vi "main_copy.vi"() -> ()   [LabVIEW 2017]
uses:
  <vilib>/DAQmx/write.llb/DAQmx Write (Digital Bool 1Line 1Point).vi
  <vilib>/DAQmx/read.llb/DAQmx Read (Counter U32 1Chan 1Samp).vi
  <vilib>/DAQmx/write.llb/DAQmx Write (Digital 1D Bool 1Chan 1Samp).vi
  <vilib>/DAQmx/create/channels.llb/DAQmx Create Channel (CI-Count Edges).vi
  <vilib>/DAQmx/miscellaneous.llb/DAQmx Fill In Error Info.vi
  <vilib>/DAQmx/create/channels.llb/DAQmx Create Channel (DO-Digital Output).vi
  <resource>/objmgr/daqmx.rc
panel:
  in  "Digital real/sham stim channels":tag="PCI-DAQ/port0/line3, PCI-DAQ/port0/line7"
  in  "Analog pulse channel":tag="PCI-DAQ/ao0"
  in  "OEP sample clock in":tag="/PCI-DAQ/PFI0"
  in  "Onboard counter":tag="PCI-DAQ/ctr1"
  in  "DAQ probe channel":tag="PCI-DAQ/port0/line5"
  out "Learning rate (for adaptive threshold)":dbl(graph)=0.005000000792214087
  out "Phase threshold":sgl(graph)=145.96965
  in  "Stim even when\ntarget exceeded":bool=TRUE
  in  "Sham stimulations:":i32=1 min=0
  in  "Real stimulations:":i32=1 min=1
  out "Stim time":i64
  out "Crossing time":i64
  out "Crossing level":sgl
  out "Time on (samp.)":i64
  out "Clock offset":i64
  in  "probe channel":u16=8 min=1 max=8
  in  "event channel":u16=5 min=1 max=8
  in  "event port":u16=5558
  out "New event":bool
  in  "Max target":i64 min=0
  in  "Limit target":bool
  in  "Target delay":i64
  in  "Adapt target":bool
  out "Phase offset (deg.)":dbl
  in  "Avg signal freq (Hz)":dbl=6.0
  in  "Sample rate":dbl=30000.0
  in  "Stim enabled":bool
  out "OEP to LV delay":i64(graph)=235
  in  "Stop":bool
  # "FOR USE WHEN DOING 2 (OR...MORE?) CL TESTS SIMULTANEOUSLY.\nIf there are any major changes to main.vi, make sure to update this copy as well.\nYou can either use this along with main.vi, or make another copy of this with another name, but if you use main.vi, make sure to\ndisable all the analog out stuff as it is in here. Either way you also have to disable the analog out channel creation in PrepareChannels_v2.vi.\nOutputting on 2 analog channels at once with separate sample clocks isn't possible (with our DAQ).\nMake sure other channels also don't conflict between the two instances, except the sample clock in can be the same."
  # "*** Start OpenEphys acquisition before the VI. ***"
  # "*** In the audio settings in the OpenEphys GUI, reduce the buffer size to get a 10 ms buffer period.  If ASIO is installed and enabled in\nthe Open Ephys build, use ASIO with sample rate (in audio settings) = 192,000 Hz and buffer size = 192 (1 ms buffer period). ***"
  # "Inputs"
  # "Delay control"
  # "Stim pattern if enabled"
  # "Event info"
  # "Threshold estimation"
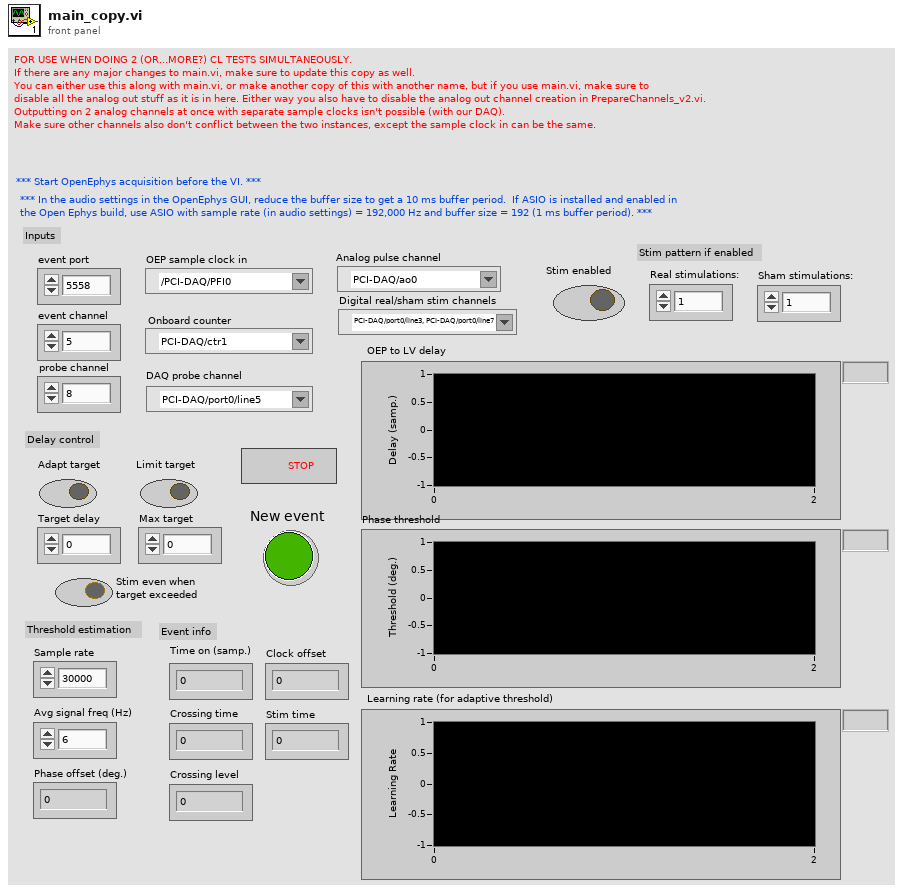
[diagram p1: front panel]
types:
  T1 = typedef "Rendezvous RefNum" = refnum<k1>
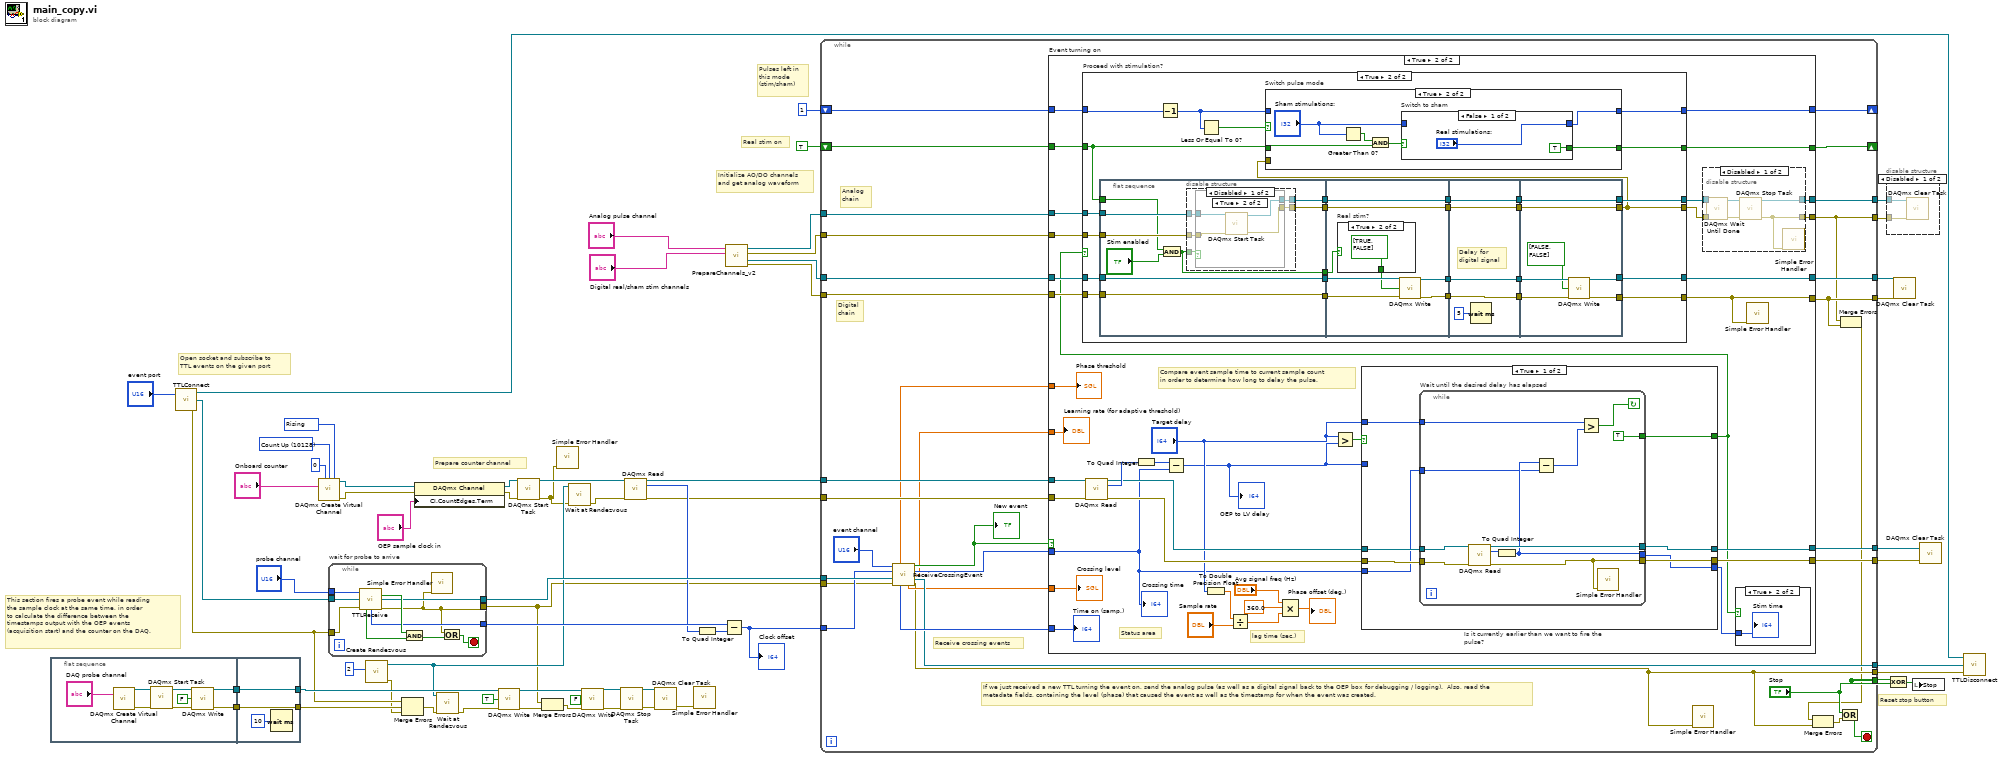
[diagram p0: block diagram]
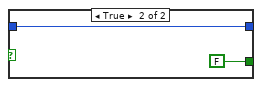
[diagram p8: hidden frame]
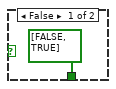
[diagram p11: hidden frame]
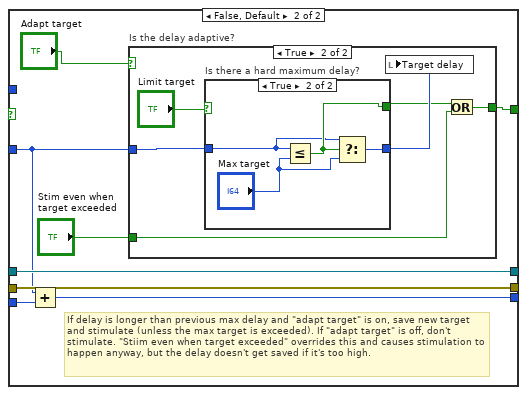
[diagram p12: hidden frame]
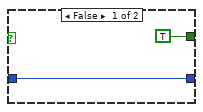
[diagram p14: hidden frame]
diagram:
  w48 = 10280 items=["Rising"=10280, "Falling"=10171] ("edge")
  w49 = 10128 items=["Count Up"=10128, "Count Down"=10124, "Externally Controlled"=10326] ("count direction")
  # "Pulses left in \nthis mode\n(stim/sham)"
  # "Real stim on"
  # "Reset stop button"
  # "This section fires a probe event while reading\nthe sample clock at the same time, in order\nto calculate the difference between the \ntimestamps output with the OEP events\n(acquisition start) and the counter on the DAQ."
  # "Prepare counter channel"
  # "Initialize AO/DO channels\nand get analog waveform"
  # "Open socket and subscribe to\nTTL events on the given port"
  n1 = flat-sequence {
    tunnel: [w66] -> w31
    tunnel: [w64] -> w30
    tunnel: [w72] -> w21
    tunnel: [w73] -> w28
    tunnel: w31 -> [w73]
    tunnel: w30 -> [w72]
    frame #0 {
      n2 = call-poly <vilib>:"DAQmx Create Virtual Channel.vi"("lines"="DAQ probe channel") -> ("task out"=w69:refnum<k21>, "error out"=w70:errorcluster)  [unwired: 13 in]
      n3 = call <vilib>:"DAQmx Start Task.vi"("task/channels in"=w69, "error in"=w70) -> ("task out"=w67:refnum<k21>, "error out"=w65:errorcluster)  [unwired: 12 in]
      n4 = call-poly <vilib>:"DAQmx Write.vi"("task/channels in"=w67, "data"=FALSE, "error in"=w65) -> ("task out"=w66:refnum<k21>, "error out"=w64:errorcluster)  [unwired: 10 in, 1 out]
    }
    frame #1 {
      n5 = Wait (ms)(milliseconds to wait=u32 10) -> ()  [unwired: 1 out]
    }
  }
  n6 = call "TTLConnect.vi"("port"="event port") -> ("context out"=w61:refnum<class "zmq_context.lvclass">, "socket out"=w43:refnum<class "zmq_socket.lvclass">, "error out"=w22:errorcluster)  [unwired: 1 in]
  n7 = call-poly <vilib>:"DAQmx Create Virtual Channel.vi"("initial count"=u32 0, "count direction"=w49, "edge"=w48, "counter"="Onboard counter") -> ("task out"=w51:refnum<k21>, "error out"=w50:errorcluster)  [unwired: 10 in]
  n8 = while "wait for probe to arrive" {
    tunnel: w43 -> [w83]
    tunnel: "probe channel" -> [w82]
    tunnel: [w79] -> w41
    tunnel: [w74] -> w11
    tunnel: [w78] -> w32
    tunnel: w22 -> [w77]
    stop <- w76 stop-if-true
    n9 = call "TTLReceive.vi"("channel"=w82, "socket in"=w83, "error in"=w77) -> ("new TTL"=w81:bool, "socket out"=w78:refnum<class "zmq_socket.lvclass">, "event on"=w80:bool, "timestamp"=w79:i64, "error out"=w74:errorcluster)  [unwired: 6 in, 2 out]
    n10 = And(x=w81, y=w80) -> (x .and. y?=w75:bool)
    n11 = call <vilib>:"Simple Error Handler.vi"("error in (no error)"=w74) -> ()  [unwired: 4 in, 5 out]
    n12 = Or(x=w74, y=w75) -> (x .or. y?=w76:bool)
  }
  n13 = call <vilib>:"Create Rendezvous.vi"("size (2)"=2) -> ("error out"=w14:errorcluster, "rendezvous"=w20:T1)  [unwired: 4 in, 1 out]
  n14 = Merge Errors(w22, w21, w14) -> (w19:errorcluster)
  n15 = property class="DAQmx Channel"(reference=w51, error in=w50, "CI.CountEdges.Term"="OEP sample clock in") -> (reference out=w47:refnum<k21>, error out=w46:errorcluster)
  n16 = call <vilib>:"Wait at Rendezvous.vi"("error in (no error)"=w19, "rendezvous"=w20) -> ("error out"=w18:errorcluster)  [unwired: 3 in, 2 out]
  n17 = call-poly <vilib>:"DAQmx Write.vi"("task/channels in"=w28, "data"=TRUE, "error in"=w18) -> ("task out"=w27:refnum<k21>, "error out"=w17:errorcluster)  [unwired: 10 in, 1 out]
  n18 = call <vilib>:"DAQmx Start Task.vi"("task/channels in"=w47, "error in"=w46) -> ("task out"=w39:refnum<k21>, "error out"=w2:errorcluster)  [unwired: 12 in]
  n19 = Merge Errors(w11, w17) -> (w16:errorcluster)
  n20 = call <vilib>:"Simple Error Handler.vi"("error in (no error)"=w2) -> ()  [unwired: 4 in, 5 out]
  n21 = call <vilib>:"Wait at Rendezvous.vi"("error in (no error)"=w2, "rendezvous"=w20) -> ("error out"=w23:errorcluster)  [unwired: 3 in, 2 out]
  n22 = call-poly <vilib>:"DAQmx Write.vi"("task/channels in"=w27, "data"=FALSE, "error in"=w16) -> ("task out"=w35:refnum<k21>, "error out"=w34:errorcluster)  [unwired: 10 in, 1 out]
  n23 = call <vilib>:"DAQmx Stop Task.vi"("task/channels in"=w35, "error in"=w34) -> ("task out"=w38:refnum<k21>, "error out"=w37:errorcluster)  [unwired: 12 in]
  n24 = call-poly <vilib>:"DAQmx Read.vi"("task/channels in"=w39, "error in"=w23) -> ("task out"=w12:refnum<k21>, "data"=w26:u32, "error out"=w24:errorcluster)  [unwired: 11 in]
  n25 = call <vilib>:"DAQmx Clear Task.vi"("task in"=w38, "error in"=w37) -> ("error out"=w1:errorcluster)  [unwired: 13 in]
  n26 = call <vilib>:"Simple Error Handler.vi"("error in (no error)"=w1) -> ()  [unwired: 4 in, 5 out]
  n27 = To Quad Integer(1:w26) -> (0:w29:i64)
  n28 = Subtract(x=w41, y=w29) -> (x-y=w40:i64)
  "Clock offset" <- w40
  n29 = call "PrepareChannels_v2.vi"("AO Physical channels"="Analog pulse channel", "DO Physical channels"="Digital real/sham stim channels") -> ("AO task out"=w60:refnum<k21>, "AO error out"=w57:errorcluster, "DO task out"=w59:refnum<k21>, "DO error out"=w58:errorcluster)  [unwired: 4 in, 1 out]
  n30 = while {
    tunnel: w11 -> [w103]
    tunnel: [w86] -> w52
    tunnel: w32 -> [w105]
    tunnel: w60 -> [w115]
    tunnel: w59 -> [w114]
    tunnel: w58 -> [w113]
    tunnel: w57 -> [w108]
    tunnel: [w106] -> w4
    tunnel: [w85] -> w3
    tunnel: [w112] -> w56
    tunnel: [w87] -> w55
    tunnel: ["Stop"] -> w54
    tunnel: w12 -> [w111]
    tunnel: [w110] -> w45
    tunnel: [w109] -> w44
    tunnel: w40 -> [w104]
    tunnel: w24 -> [w107]
    tunnel: [w99] -> w13
    shift-right: [w93] -> _
    shift-left: TRUE -> [w95]
    shift-right: [w94] -> _
    shift-left: 1 -> [w96]
    stop <- w90 stop-if-true
    # "Analog \nchain"
    # "Digital\nchain"
    # "If we just received a new TTL turning the event on, send the analog pulse (as well as a digital signal back to the OEP box for debugging / logging).  Also, read the metadata fields, containing the level (phase) that caused the event as well as the timestamp for when the event was created."
    # "Receive crossing events"
    n31 = call "ReceiveCrossingEvent.vi"("channel"="event channel", "clock offset"=w104, "socket in"=w105, "error in"=w103) -> ("threshold"=w92:sgl, "new crossing"=w102:bool, "crossing time"=w101:i64, "learning rate"=w91:dbl, "socket out"=w99:refnum<class "zmq_socket.lvclass">, "event time"=w100:i64, "crossing level"=w98:sgl, "error out"=w86:errorcluster)  [unwired: 3 in, 1 out]
    "New event" <- w102
    n32 = case "Event turning on" shown="True" w102 {
      tunnel: w115 -> [w123 w157]
      tunnel: w108 -> [w122 w156]
      tunnel: [w123 w148] -> w106
      tunnel: [w122 w125] -> w85
      tunnel: w114 -> [w121 w160]
      tunnel: w113 -> [w120 w158]
      tunnel: [w121 w161] -> w112
      tunnel: [w120 w124] -> w87
      tunnel: w101 -> [_ w143]
      tunnel: w111 -> [w119 w155]
      tunnel: w107 -> [w118 w152]
      tunnel: [w119 w150] -> w110
      tunnel: [w118 w149] -> w109
      tunnel: w100 -> [_ w144]
      tunnel: w98 -> [_ w138]
      tunnel: w96 -> [w117 w131]
      tunnel: w95 -> [w116 w130]
      tunnel: [w117 w129] -> w94
      tunnel: [w116 w128] -> w93
      tunnel: w92 -> [_ w127]
      tunnel: w91 -> [_ w126]
      frame False {
      }
      frame True {
        # "Status area"
        # "lag time (sec.)"
        # "Compare event sample time to current sample count\nin order to determine how long to delay the pulse."
        n33 = call-poly <vilib>:"DAQmx Read.vi"("task/channels in"=w155, "error in"=w152) -> ("task out"=w151:refnum<k21>, "data"=w154:u32, "error out"=w153:errorcluster)  [unwired: 11 in]
        n34 = To Quad Integer(1:w154) -> (0:w134:i64)
        n35 = Subtract(x=w134, y=w143) -> (x-y=w145:i64)
        "OEP to LV delay" <- w145
        n36 = To Double Precision Float(number="Target delay") -> (double precision float=w142:dbl)
        n37 = Divide(x=w142, y="Sample rate") -> (x/y=w141:dbl)
        n38 = Compound Arithmetic op=MULTIPLY("Avg signal freq (Hz)", 360.0 ("y"), w141) -> (→"Phase offset (deg.)":dbl)
        n39 = Greater?(x="Target delay", y=w145) -> (0:w159:bool)
        n40 = case "Is it currently earlier than we want to fire the pulse?" shown="True" w159 {
          tunnel: w145 -> [_ w281]
          tunnel: "Target delay" -> [w261 _]
          tunnel: w153 -> [w266 w286]
          tunnel: [w265 w286] -> w149
          tunnel: w143 -> [w260 w284]
          tunnel: w151 -> [w267 w285]
          tunnel: [w264 w285] -> w150
          tunnel: [w263 w280] -> w133
          tunnel: [w262 w283] -> w132
          frame True {
            n41 = while "Wait until the desired delay has elapsed" {
              tunnel: w267 -> [w277]
              tunnel: w266 -> [w278]
              tunnel: [w268] -> w265
              tunnel: [w276] -> w264
              tunnel: [TRUE] -> w263
              tunnel: [w271] -> w262
              tunnel: w261 -> [w272]
              tunnel: w260 -> [w270]
              stop <- w274 continue-if-true
              n42 = call-poly <vilib>:"DAQmx Read.vi"("task/channels in"=w277, "error in"=w278) -> ("task out"=w276:refnum<k21>, "data"=w273:u32, "error out"=w268:errorcluster)  [unwired: 11 in]
              n43 = To Quad Integer(1:w273) -> (0:w271:i64)
              n44 = Subtract(x=w271, y=w270) -> (x-y=w269:i64)
              n45 = Greater?(x=w272, y=w269) -> (0:w274:bool)
              n46 = call <vilib>:"Simple Error Handler.vi"("error in (no error)"=w268) -> ()  [unwired: 4 in, 5 out]
            }
          }
          frame False, Default {
            # "If delay is longer than previous max delay and \"adapt target\" is on, save new target and stimulate (unless the max target is exceeded). If \"adapt target\" is off, don't stimulate. \"Stiim even when target exceeded\" overrides this and causes stimulation to happen anyway, but the delay doesn't get saved if it's too high."
            n47 = Add(x=w281, y=w284) -> (x+y=w283:i64)
            n48 = case "Is the delay adaptive?" shown="True" "Adapt target" {
              tunnel: w281 -> [_ w292]
              tunnel: [w287 w290] -> w280
              tunnel: "Stim even when\ntarget exceeded" -> [w287 w288]
              frame False {
              }
              frame True {
                n49 = case "Is there a hard maximum delay?" shown="True" "Limit target" {
                  tunnel: [w295 w299] -> w291
                  tunnel: w292 -> [w295 w297]
                  tunnel: [TRUE w298] -> w289
                  frame False {
                  }
                  frame True {
                    n50 = Less Or Equal?(x=w297, y="Max target") -> (x <= y?=w298:bool)
                    n51 = Select(t=w297, s=w298, f="Max target") -> (s? t:f=w299:i64)
                  }
                }
                n52 = local write "Target delay"(w291) -> ()
                n53 = Or(x=w289, y=w288) -> (x .or. y?=w290:bool)
              }
            }
          }
        }
        n54 = case "Proceed with stimulation?" shown="True" w133 {
          tunnel: [w174 w191] -> w161
          tunnel: w160 -> [w174 w190]
          tunnel: w158 -> [w173 w189]
          tunnel: w157 -> [w176 w188]
          tunnel: w156 -> [w175 w187]
          tunnel: [w173 w186] -> w124
          tunnel: [w175 w183] -> w135
          tunnel: [w176 w185] -> w147
          tunnel: w131 -> [w172 w182]
          tunnel: w130 -> [w171 w179]
          tunnel: [w172 w178] -> w129
          tunnel: [w171 w177] -> w128
          frame False {
          }
          frame True {
            n55 = flat-sequence {
              tunnel: [w224] -> w203
              tunnel: [w221] -> w202
              tunnel: [w220] -> w201
              tunnel: w189 -> [w220]
              tunnel: w190 -> [w221]
              tunnel: w187 -> [w223]
              tunnel: w188 -> [w222]
              tunnel: [w219] -> w200
              tunnel: w179 -> [w217]
              tunnel: [w216] -> w184
              tunnel: [w243] -> w199
              tunnel: [w241] -> w198
              tunnel: w203 -> [w245]
              tunnel: [w245] -> w197
              tunnel: w202 -> [w244]
              tunnel: w201 -> [w242]
              tunnel: w200 -> [w240]
              tunnel: [w240] -> w196
              tunnel: w184 -> [w239]
              tunnel: [w252] -> w195
              tunnel: w199 -> [w252]
              tunnel: [w251] -> w194
              tunnel: w198 -> [w251]
              tunnel: w197 -> [w249]
              tunnel: [w249] -> w193
              tunnel: w196 -> [w248]
              tunnel: [w248] -> w192
              tunnel: [w258] -> w191
              tunnel: w195 -> [w259]
              tunnel: w194 -> [w257]
              tunnel: [w256] -> w186
              tunnel: w193 -> [w255]
              tunnel: [w255] -> w185
              tunnel: [w254] -> w183
              tunnel: w192 -> [w254]
              frame #0 {
                n56 = And(x=w217, y="Stim enabled") -> (x .and. y?=w216:bool)
                n57 = disable-structure shown="Disabled" {
                  disable-tunnel: [w229 w237] -> w224
                  disable-tunnel: w223 -> [w228 w236]
                  disable-tunnel: w222 -> [w227 w237]
                  disable-tunnel: [w226 w236] -> w219
                  disable-tunnel: w216 -> [w225 _]
                  frame Disabled {
                    n58 = case shown="True" w225 {
                      tunnel: [w231 w235] -> w229
                      tunnel: w228 -> [w230 w234]
                      tunnel: w227 -> [w231 w233]
                      tunnel: [w230 w232] -> w226
                      frame False {
                      }
                      frame True {
                        n59 = call <vilib>:"DAQmx Start Task.vi"("task/channels in"=w233, "error in"=w234) -> ("task out"=w235:refnum<k21>, "error out"=w232:errorcluster)  [unwired: 12 in]
                      }
                    }
                  }
                  frame Enabled {
                  }
                }
              }
              frame #1 {
                n60 = case "Real stim?" shown="True" w239 {
                  tunnel: [bool[] [FALSE, TRUE] ("data") bool[] [TRUE, FALSE] ("data")] -> w238
                  frame False {
                  }
                  frame True {
                  }
                }
                n61 = call-poly <vilib>:"DAQmx Write.vi"("task/channels in"=w244, "data"=w238, "error in"=w242) -> ("task out"=w243:refnum<k21>, "error out"=w241:errorcluster)  [unwired: 10 in, 1 out]
              }
              frame #2 {
                # "Delay for \ndigital signal"
                n62 = Wait (ms)(milliseconds to wait=u32 5) -> ()  [unwired: 1 out]
              }
              frame #3 {
                n63 = call-poly <vilib>:"DAQmx Write.vi"("task/channels in"=w259, "data"=bool[] [FALSE, FALSE], "error in"=w257) -> ("task out"=w258:refnum<k21>, "error out"=w256:errorcluster)  [unwired: 10 in, 1 out]
              }
            }
            n64 = Decrement(x=w182) -> (x-1=w180:i32)
            n65 = Less Or Equal To 0?(x=w180) -> (x <= 0?=w181:bool)
            n66 = case "Switch pulse mode" shown="True" w181 {
              tunnel: w183 -> [_ _]
              tunnel: w180 -> [w205 _]
              tunnel: w179 -> [w204 w210]
              tunnel: [w205 w207] -> w178
              tunnel: [w204 w206] -> w177
              frame False {
              }
              frame True {
                n67 = Greater Than 0?(x="Sham stimulations:") -> (x > 0?=w211:bool)
                n68 = And(x=w211, y=w210) -> (x .and. y?=w209:bool)
                n69 = case "Switch to sham" shown="False" w209 {
                  tunnel: "Sham stimulations:" -> [_ w215]
                  tunnel: ["Real stimulations:" w215] -> w207
                  tunnel: [TRUE FALSE] -> w206
                  frame False {
                  }
                  frame True {
                  }
                }
              }
            }
          }
        }
        n70 = disable-structure shown="Disabled" {
          disable-tunnel: [w165 w169] -> w148
          disable-tunnel: w147 -> [w164 w169]
          disable-tunnel: w135 -> [w163 w168]
          disable-tunnel: [w162 w168] -> w125
          frame Disabled {
            n71 = call <vilib>:"DAQmx Wait Until Done.vi"("task/channels in"=w164, "error in"=w163) -> ("task out"=w166:refnum<k21>, "error out"=w167:errorcluster)  [unwired: 12 in]
            n72 = call <vilib>:"DAQmx Stop Task.vi"("task/channels in"=w166, "error in"=w167) -> ("task out"=w165:refnum<k21>, "error out"=w162:errorcluster)  [unwired: 12 in]
            n73 = call <vilib>:"Simple Error Handler.vi"("error in (no error)"=w162) -> ()  [unwired: 4 in, 5 out]
          }
          frame Enabled {
          }
        }
        n74 = case shown="True" w133 {
          tunnel: w132 -> [_ w170]
          frame False {
          }
          frame True {
            "Stim time" <- w170
          }
        }
        n75 = call <vilib>:"Simple Error Handler.vi"("error in (no error)"=w124) -> ()  [unwired: 4 in, 5 out]
        "Time on (samp.)" <- w144
        "Crossing time" <- w143
        "Crossing level" <- w138
        "Phase threshold" <- w127
        "Learning rate (for adaptive threshold)" <- w126
      }
    }
    n76 = call <vilib>:"Simple Error Handler.vi"("error in (no error)"=w86) -> ()  [unwired: 4 in, 5 out]
    n77 = Merge Errors(w85, w87) -> (w84:errorcluster)
    n78 = Merge Errors(w84, w86) -> (w88:errorcluster)
    n79 = Or(x="Stop", y=w88) -> (x .or. y?=w90:bool)
  }
  n80 = disable-structure shown="Disabled" {
    disable-tunnel: w4 -> [w301 _]
    disable-tunnel: w3 -> [w300 _]
    frame Disabled {
      n81 = call <vilib>:"DAQmx Clear Task.vi"("task in"=w301, "error in"=w300) -> ()  [unwired: 13 in, 1 out]
    }
    frame Enabled {
    }
  }
  n82 = Exclusive Or(1:w54, 2:w54) -> (0:w53:bool)
  n83 = call <vilib>:"DAQmx Clear Task.vi"("task in"=w56, "error in"=w55) -> ()  [unwired: 13 in, 1 out]
  n84 = local write "Stop"(w53) -> ()
  n85 = call <vilib>:"DAQmx Clear Task.vi"("task in"=w45, "error in"=w44) -> ()  [unwired: 13 in, 1 out]
  n86 = call "TTLDisconnect.vi"("error in"=w52, "socket in"=w13, "context in"=w61) -> ()  [unwired: 1 in, 1 out]
